vi "ReadValuesOfMoreTransmitters.vi"() -> ()   [LabVIEW 2014]
uses:
  K_S30c_dll.lvlib
panel:
  in  "Time [ms]":u32
  in  "clear Log":bool
  in  "Start / Stop":bool
  in  "Stop":bool
  in  "Log":string
  out "values":sgl[](array[numeric])
  out "communication":bool[](array[boolean])
  out "error out":errorcluster
  in  "Devices":T1(array[cluster])=[{"Address"=1, "Channel"=enum."P1"}, {"Address"=1, "Channel"=enum."TOB1"}, {"Address"=2, "Channel"=enum."P1"}]
  # "simple demonstation how to read out values from n devices"
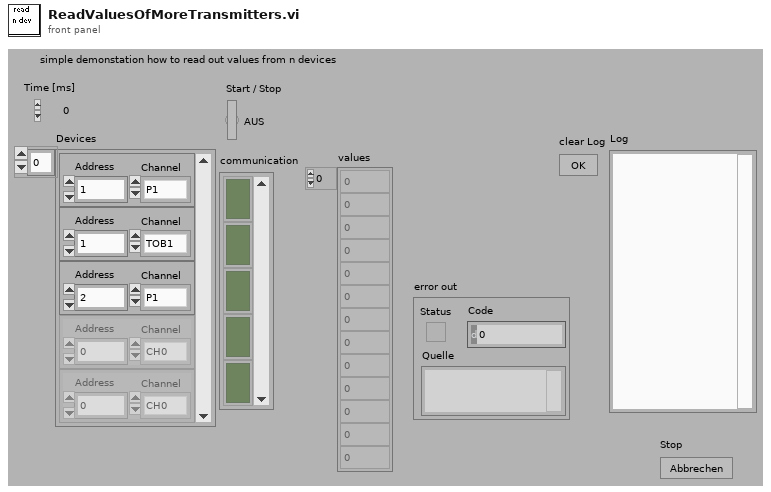
[diagram p1: front panel]
types:
  T1 = cluster{"Address":u8, "Channel":enum16{"CH0", "P1", "P2", "T", "TOB1", "TOB2"}}[]
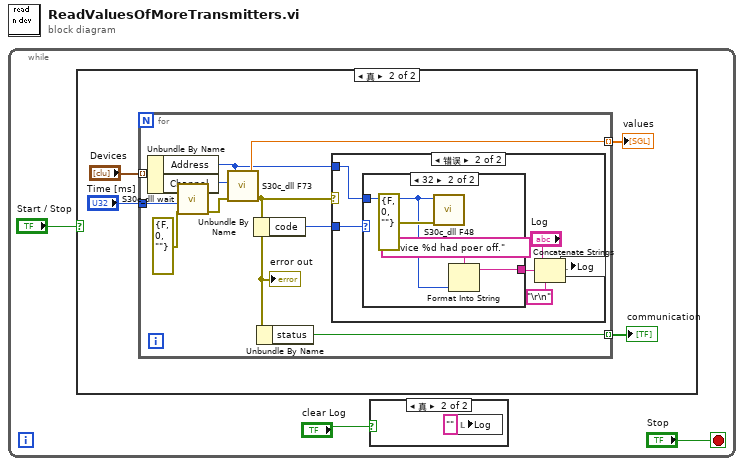
[diagram p0: block diagram]
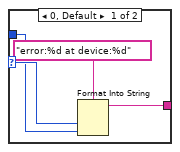
[diagram p5: hidden frame]
diagram:
  n1 = while {
    stop <- "Stop" stop-if-true
    n2 = case shown="真" "Start / Stop" {
      frame False {
      }
      frame True {
        n3 = for {
          tunnel: "Devices" -> [w18] mode=indexing
          tunnel: [w15] -> w7 mode=indexing
          tunnel: [w12] -> w6 mode=indexing
          tunnel: "Time [ms]" -> [w10]
          n4 = Unbundle By Name(w18) -> ("Address"=w14:u8, "Channel"=w16:enum16{"CH0", "P1", "P2", "T", "TOB1", "TOB2"})
          n5 = call "S30c_dll wait.vi"("error in (no error)"=errorcluster {"status"=FALSE, "code"=0, "source"=""}, "Time [ms]"=w10) -> ("error out"=w11:errorcluster)  [unwired: 5 in]
          n6 = call "S30c_dll F73.vi"("error in"=w11, "Channel"=w16, "Dev Addr"=w14) -> ("error out"=w13:errorcluster, "Value"=w15:sgl)  [unwired: 2 in, 1 out]
          "error out" <- w13
          n7 = Unbundle By Name(w13) -> ("code"=w17:i32)
          n8 = Unbundle By Name(w13) -> ("status"=w12:bool)
          n9 = case shown="错误" w13 {
            tunnel: w17 -> [_ w24]
            tunnel: w14 -> [_ w19]
            frame No Error {
            }
            frame Error {
              n10 = case shown="32" w24 {
                selector: w24 -> [w27 _]
                tunnel: [w26 w30] -> w22
                tunnel: w19 -> [w25 w29]
                frame 0, Default {
                  n11 = Format Into String(format string="error:%d at device:%d" ("Format-String"), w27, w25) -> (resulting string=w26:string)  [unwired: 2 in, 1 out]
                }
                frame 32 {
                  n12 = call "S30c_dll F48.vi"("error in"=errorcluster {"status"=FALSE, "code"=0, "source"=""}, "Dev Addr"=w29) -> ()  [unwired: 3 in, 3 out]
                  n13 = Format Into String(format string="device %d had poer off." ("Format-String"), w29) -> (resulting string=w30:string)  [unwired: 2 in, 1 out]
                }
              }
              n14 = Concatenate Strings("Log", w22, "\r\n") -> (w21:string)
              n15 = local write "Log"(w21) -> ()
            }
          }
        }
        "communication" <- w6
        "values" <- w7
      }
    }
    n16 = case shown="真" "clear Log" {
      frame False {
      }
      frame True {
        n17 = local write "Log"("" ("Log")) -> ()
      }
    }
  }
